vi "macro_BoolCmd_Send_OnEdge.vi"() -> ()   [LabVIEW 2019, in "Trajectory_Library.lvlib"]
uses:
  Trajectory_Library.lvlib
  VI/DigSeqLogic_Edge_On.vi
  VI/BoolCmd_Send_Internal.vi
  VI/BoolCmd_ObtainQueue.vi
panel:
  in  "Button":bool
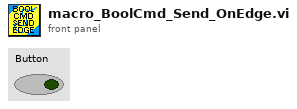
[diagram p1: front panel]
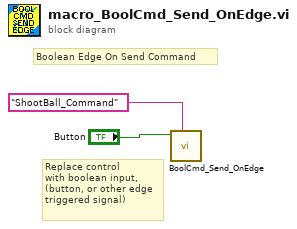
[diagram p0: block diagram]
diagram:
  # "Boolean Edge On Send Command"
  # "Replace control\nwith boolean input,\n(button, or other edge\ntriggered signal)"
  n1 = call "BoolCmd_Send_OnEdge.vi"("Command Name"="ShootBall_Command", "Value"="Button") -> ()  [unwired: 9 in, 1 out]
